vi "Read Results from processing.vi"(8 "error in":errorcluster, 11 "Temperature Chamber Model runtime in":refnum<class "Temperature Chamber Model runtime.lvclass">) -> (0 "error out":errorcluster, 2 "Results from processing":T1, 3 "Temperature Chamber Model runtime out":refnum<class "Temperature Chamber Model runtime.lvclass">)   [LabVIEW 2015, in "Temperature Chamber Model runtime.lvclass"]
uses:
  Temperature Chamber Model runtime.lvclass
  configuration/result data indices.ctl
  Temperature Chamber Model runtime.lvclass/Temperature Chamber Model runtime.ctl
  configuration/Temperature Chamber Model configuration.lvclass
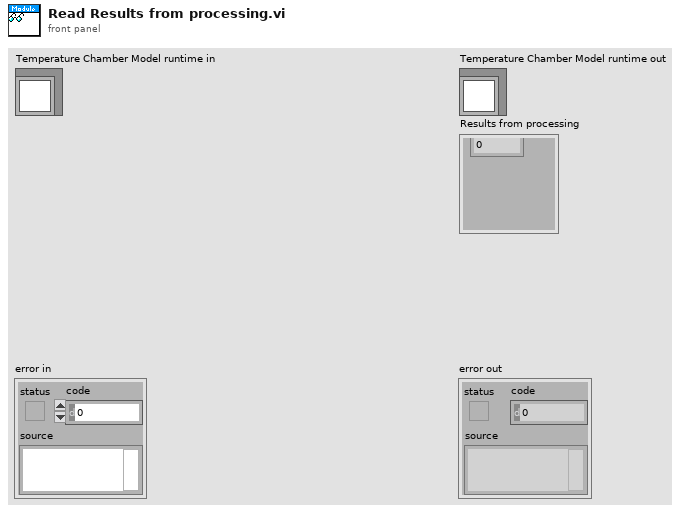
[diagram p1: front panel]
types:
  T1 = typedef "Temperature Chamber Model configuration.lvclass/result data indices.ctl" = cluster{"Double.Thermocouple Reading":i32}
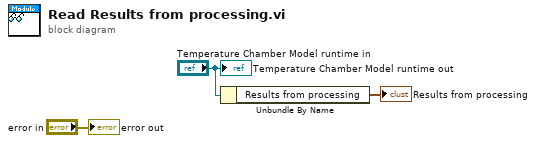
[diagram p0: block diagram]
diagram:
  n1 = Unbundle By Name("Temperature Chamber Model runtime in") -> ("Results from processing"=→"Results from processing":T1)
  "error out" <- "error in"
  "Temperature Chamber Model runtime out" <- "Temperature Chamber Model runtime in"
